vi "Read Variable.vi"(8 "error in (no error)":errorcluster, 10 "Variable Name":string, 11 "gScript Interpreter in":refnum<class "gScript Interpreter.lvclass">) -> (0 "error out":errorcluster, 2 "Memory Cell":T1, 3 "gScript Interpreter out":refnum<class "gScript Interpreter.lvclass">)   [LabVIEW 2017, in "gScript Interpreter.lvclass"]
uses:
  gScript Interpreter.lvclass
  Type Definitions/Memory Cell.ctl
  Type Definitions/Memory Cell Type Enum.ctl
  gScript Interpreter.lvclass/gScript Interpreter.ctl
  <vilib>/Utility/error.llb/Error Cluster From Error Code.vi
  <vilib>/ErrorRing/Error Ring.xnode
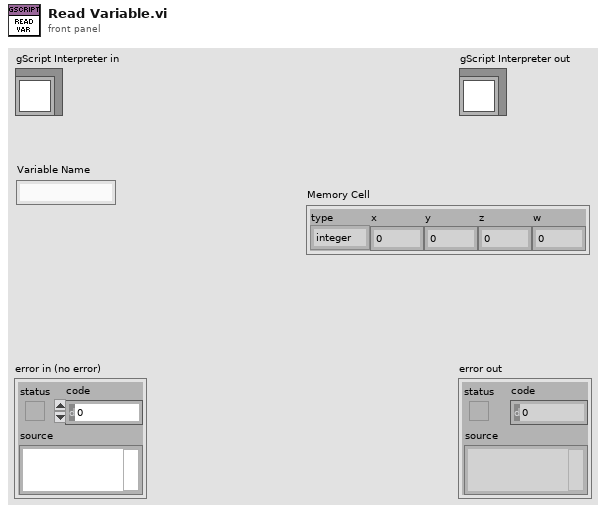
[diagram p1: front panel]
types:
  T1 = typedef "Memory Cell.ctl" = cluster{"type":T2, "x":dbl, "y":dbl, "z":dbl, "w":dbl}
  T2 = typedef "Memory Cell Type Enum.ctl" = enum16{"integer", "float", "vector", "rotation"}
  T3 = typedef "Stack Frame.ctl" = cluster{"Variable Table":T4}
  T4 = typedef "Variable Table.ctl" = T5[]
  T5 = typedef "Variable.ctl" = cluster{"Variable Name":string, "Memory Cell":T1}
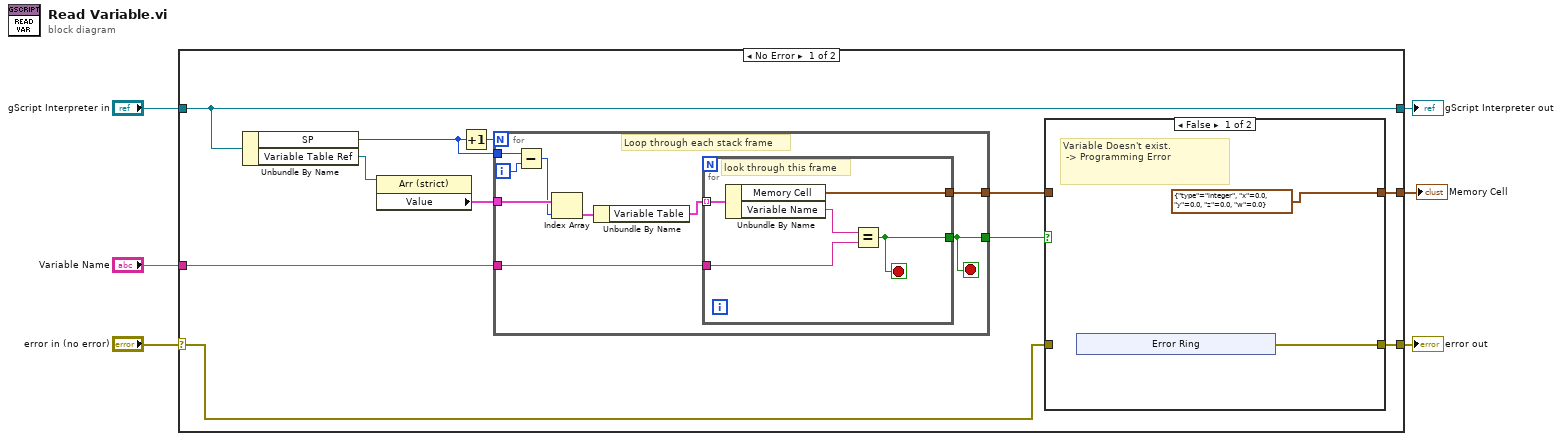
[diagram p0: block diagram]
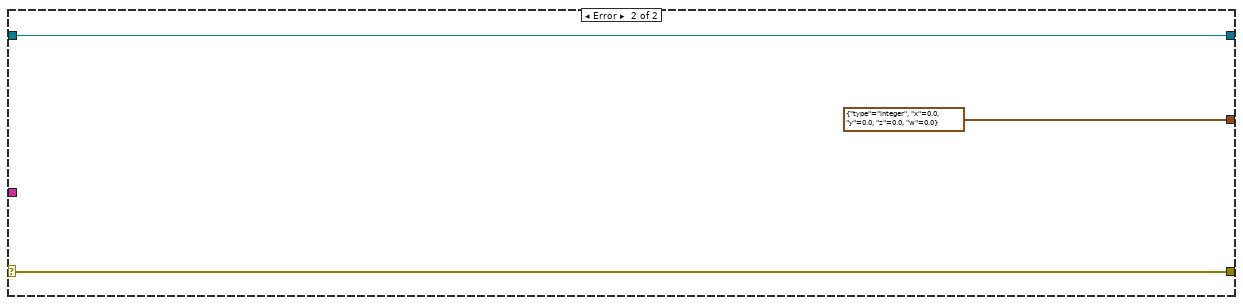
[diagram p3: hidden frame]
diagram:
  n1 = case shown="No Error" "error in (no error)" {
    selector: "error in (no error)" -> [w10 w42]
    tunnel: [w11 w42] -> w5
    tunnel: [w17 w41] -> w3
    tunnel: "gScript Interpreter in" -> [w17 w41]
    tunnel: "Variable Name" -> [w15 _]
    tunnel: [w12 T1 {"type"=enum."integer", "x"=0.0, "y"=0.0, "z"=0.0, "w"=0.0} ("Memory Cell")] -> w1
    frame No Error {
      n2 = Unbundle By Name(w17) -> ("SP"=w7:i32, "Variable Table Ref"=w9:refnum<vi>)
      n3 = property class="Arr (strict)"(reference=w9) -> ("Value"=w16:T3[])  [unwired: 1 in, 2 out]
      n4 = Increment(x=w7) -> (x+1=w8:i32)
      n5 = for {
        N: w8 -> [_]
        tunnel: w16 -> [w24]
        tunnel: w15 -> [w26]
        tunnel: [w21] -> w14
        tunnel: [w25] -> w13
        tunnel: w7 -> [w18]
        i -> [w23]
        stop <- w21 stop-if-true
        # "Loop through each stack frame"
        n6 = Subtract(x=w18, y=w23) -> (x-y=w22:i32)
        n7 = Index Array(array=w24, index=w22) -> (element=w20:T3)
        n8 = Unbundle By Name(w20) -> ("Variable Table"=w19:T4)
        n9 = for {
          tunnel: w19 -> [w31] mode=indexing
          tunnel: w26 -> [w29]
          tunnel: [w28] -> w21
          tunnel: [w27] -> w25
          stop <- w28 stop-if-true
          # "look through this frame"
          n10 = Unbundle By Name(w31) -> ("Memory Cell"=w27:T1, "Variable Name"=w30:string)
          n11 = Equal?(x=w30, y=w29) -> (x = y?=w28:bool)
        }
      }
      n12 = case shown="False" w14 {
        tunnel: w13 -> [_ w39]
        tunnel: [T1 {"type"=enum."integer", "x"=0.0, "y"=0.0, "z"=0.0, "w"=0.0} ("Memory Cell") w39] -> w12
        tunnel: w10 -> [_ w38]
        tunnel: [w32 w38] -> w11
        frame False {
          # "Variable Doesn't exist.\n -> Programming Error"
          n13 = xnode "Error Ring"() -> ("error out"=w32:errorcluster)
        }
        frame True {
          # "Variable Exists so Return it"
        }
      }
    }
    frame Error {
    }
  }
  "error out" <- w5
  "gScript Interpreter out" <- w3
  "Memory Cell" <- w1
